vi "ArmControl.vi"   [LabVIEW 2012]
uses:
  State_Machine_Enum.ctl
  <vilib>/Rock Robotics/WPI/Relay/WPI_RelayValue.ctl
  Robot Global Data.vi
types:
  T1 = typedef "State_Machine_Enum.ctl" = enum16{"Idle", "Start", "Do", "Stop", "Init"}
  T2 = typedef "WPI_RelayValue.ctl" = enum16{"Off", "On", "Forward", "Reverse"}
  T3 = typedef "LoopDisable.ctl" = cluster{"Climb.vi":bool, "LauncherAngle.vi":bool, "Launcher.vi":bool, "ArmControl.vi":bool, "WinchMotor.vi":bool}
  T4 = typedef "WPI_RelayDevRef.ctl" = cluster{"DevStatus":errorcluster, "Relay Channel":T5, "Digital Module":T6, "Relay Direction":T7}
  T5 = typedef "FPGA_DIORelayChannel.ctl" = enum8{"Relay 1", "Relay 2", "Relay 3", "Relay 4", "Relay 5", "Relay 6", "Relay 7", "Relay 8", "Invalid"}
  T6 = typedef "FPGA_TypedefDigitalModule.ctl" = enum16{"Digital Module 1", "Digital Module 2"}
  T7 = typedef "WPI_RelayDirection.ctl" = enum16{"Both directions", "Forward only", "Reverse only"}
  T8 = typedef "WPI_DigitalInputDevRef.ctl" = cluster{"DevStatus":errorcluster, "DIO Channel":T9, "Digital Module":T6}
  T9 = typedef "FPGA_DIOChannel.ctl" = enum8{"DIO 1", "DIO 2", "DIO 3", "DIO 4", "DIO 5", "DIO 6", "DIO 7", "DIO 8", "DIO 9", "DIO 10", "DIO 11", "DIO 12", "DIO 13", "DIO 14", "Invalid"}
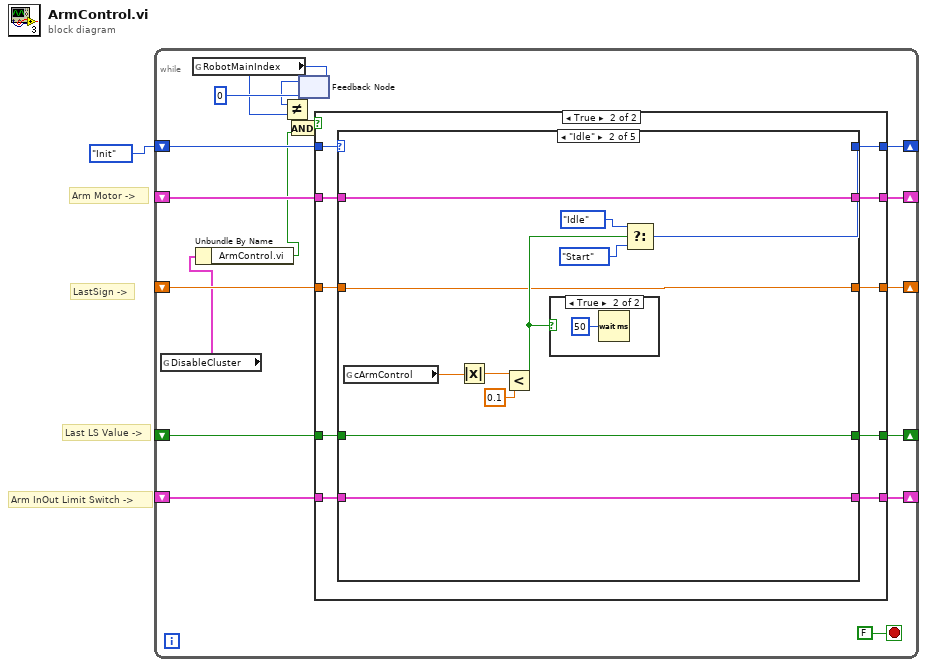
[diagram p0: block diagram]
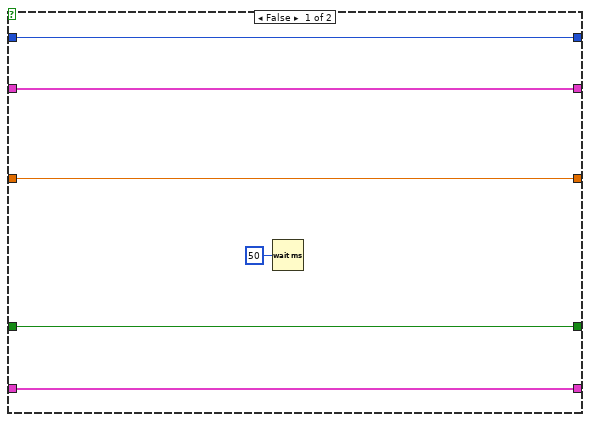
[diagram p2: hidden frame]
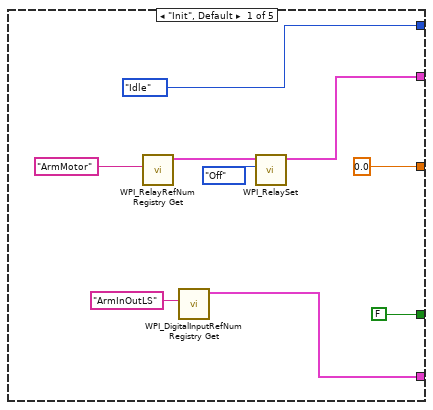
[diagram p3: hidden frame]
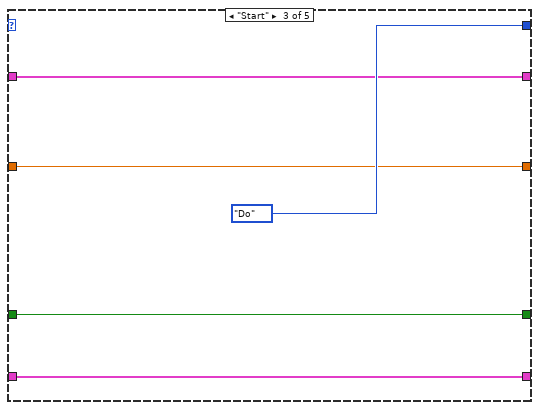
[diagram p5: hidden frame]
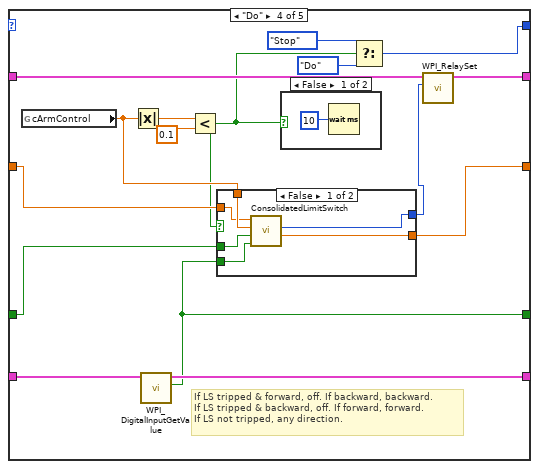
[diagram p6: hidden frame]
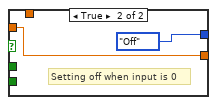
[diagram p7: hidden frame]
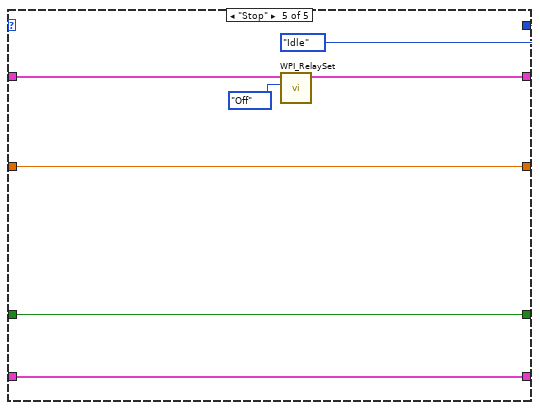
[diagram p9: hidden frame]
diagram:
  # "Last LS Value ->"
  # "LastSign ->"
  # "Arm InOut Limit Switch ->"
  # "Arm Motor ->"
  n1 = while {
    shift-right: [w18] -> _
    shift-left: _ -> [w17]
    shift-right: [w15] -> _
    shift-left: State_Machine_Enum."Init" ("State") -> [w16]
    shift-right: [w14] -> _
    shift-left: _ -> [w13]
    shift-right: [w12] -> _
    shift-left: _ -> [w11]
    shift-right: [w10] -> _
    shift-left: _ -> [w9]
    stop <- FALSE stop-if-true
    n2 = global read "Robot Global Data.vi" "DisableCluster"() -> (w2:T3)
    n3 = global read "Robot Global Data.vi" "RobotMainIndex"() -> (w7:i32)
    n4 = Unbundle By Name(w2) -> ("ArmControl.vi"=w3:bool)
    n5 = feedback #1(0 ("TeleopIndex")) -> (w6:i32)
    n6 = Not Equal?(x=w6, y=w7) -> (x != y?=w5:bool)
    n7 = And(x=w5, y=w3) -> (x .and. y?=w4:bool)
    n8 = feedback-in #1(w7) -> ()
    n9 = case shown="True" w4 {
      tunnel: [w23 w35] -> w18
      tunnel: w17 -> [w23 w34]
      tunnel: w16 -> [w20 w33]
      tunnel: [w20 w32] -> w15
      tunnel: [w21 w31] -> w14
      tunnel: w13 -> [w21 w30]
      tunnel: [w24 w29] -> w12
      tunnel: w11 -> [w24 w28]
      tunnel: [w22 w27] -> w10
      tunnel: w9 -> [w22 w26]
      frame False {
        n10 = Wait (ms)(milliseconds to wait=u32 50) -> ()  [unwired: 1 out]
      }
      frame True {
        n11 = case shown="\"Idle\"" w33 {
          tunnel: [w44 w50 w60 w77 w92] -> w35
          tunnel: w34 -> [_ w50 w60 w76 w92]
          tunnel: [State_Machine_Enum."Idle" ("State") w51 State_Machine_Enum."Do" ("f") w71 State_Machine_Enum."Idle" ("State")] -> w32
          tunnel: [w37 w47 w59 w69 w89] -> w31
          tunnel: w30 -> [_ w47 w59 w70 w90]
          tunnel: [FALSE w45 w57 w63 w88] -> w29
          tunnel: w28 -> [_ w45 w57 w64 w88]
          tunnel: [0.0 w46 w58 w66 w87] -> w27
          tunnel: w26 -> [_ w46 w58 w65 w87]
          frame "Init", Default {
            n12 = call <vilib>:"WPI_RelayRefNum Registry Get.vi"("refnum name"="ArmMotor") -> ("RelayDevRef"=w40:T4)  [unwired: 9 in, 1 out]
            n13 = call <vilib>:"WPI_DigitalInputRefNum Registry Get.vi"("refnum name"="ArmInOutLS") -> ("DigitalInputDevRef"=w44:T8)  [unwired: 9 in, 1 out]
            n14 = call <vilib>:"WPI_RelaySet.vi"("RelayValue"=WPI_RelayValue."Off", "RelayDevRef"=w40) -> ("RelayDevRef"=w37:T4)  [unwired: 8 in, 1 out]
          }
          frame "Idle" {
            n15 = global read "Robot Global Data.vi" "cArmControl"() -> (w55:dbl)
            n16 = Absolute Value(x=w55) -> (abs(x)=w54:dbl)
            n17 = Less?(x=w54, y=0.1) -> (x < y?=w48:bool)
            n18 = case shown="True" w48 {
              frame False {
              }
              frame True {
                n19 = Wait (ms)(milliseconds to wait=u32 50) -> ()  [unwired: 1 out]
              }
            }
            n20 = Select(t=State_Machine_Enum."Idle" ("f"), s=w48, f=State_Machine_Enum."Start") -> (s? t:f=w51:T1)
          }
          frame "Start" {
          }
          frame "Do" {
            # "If LS tripped & forward, off. If backward, backward.\nIf LS tripped & backward, off. If forward, forward.\nIf LS not tripped, any direction."
            n21 = global read "Robot Global Data.vi" "cArmControl"() -> (w68:dbl)
            n22 = Absolute Value(x=w68) -> (abs(x)=w75:dbl)
            n23 = call <vilib>:"WPI_DigitalInputGetValue.vi"("DigitalInputDevRef"=w76) -> ("Value"=w63:bool, "DigitalInputDevRef"=w77:T8)  [unwired: 8 in, 1 out]
            n24 = Less?(x=w75, y=0.1) -> (x < y?=w62:bool)
            n25 = case shown="False" w62 {
              tunnel: w68 -> [w83 _]
              tunnel: [w82 WPI_RelayValue."Off" ("RelayValue")] -> w67
              tunnel: [w81 w85] -> w66
              tunnel: w65 -> [w80 w85]
              tunnel: w64 -> [w79 _]
              tunnel: w63 -> [w78 _]
              frame False {
                n26 = call "ConsolidatedLimitSwitch.vi"("CurrentLSValue"=w78, "LastLSValue"=w79, "CurrentInput"=w83, "LastSign"=w80) -> ("NewSign"=w81:dbl, "RelayValue"=w82:T2)  [unwired: 6 in]
              }
              frame True {
                # "Setting off when input is 0"
              }
            }
            n27 = case shown="False" w62 {
              frame False {
                n28 = Wait (ms)(milliseconds to wait=u32 10) -> ()  [unwired: 1 out]
              }
              frame True {
              }
            }
            n29 = Select(t=State_Machine_Enum."Stop" ("State"), s=w62, f=State_Machine_Enum."Do" ("State")) -> (s? t:f=w71:T1)
            n30 = call <vilib>:"WPI_RelaySet.vi"("RelayValue"=w67, "RelayDevRef"=w70) -> ("RelayDevRef"=w69:T4)  [unwired: 8 in, 1 out]
          }
          frame "Stop" {
            n31 = call <vilib>:"WPI_RelaySet.vi"("RelayValue"=WPI_RelayValue."Off", "RelayDevRef"=w90) -> ("RelayDevRef"=w89:T4)  [unwired: 8 in, 1 out]
          }
        }
      }
    }
  }
